vi "CSV SENDER 2 - Copy.vi"() -> ()   [LabVIEW 2021]
panel:
  out "Waveform Chart":dbl[](graph)
  out "Iteration terminal":i32
  in  "Stop 2":bool
  in  "File Path":path
  in  "Number of row to read \nat a time":i32=10000
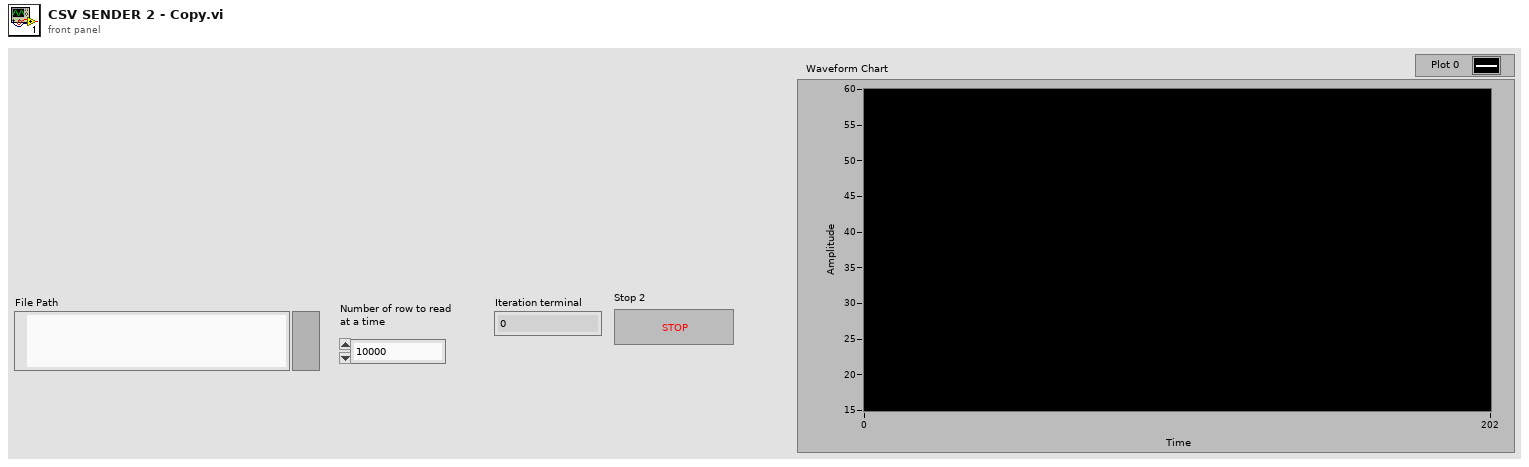
[diagram p1: front panel]
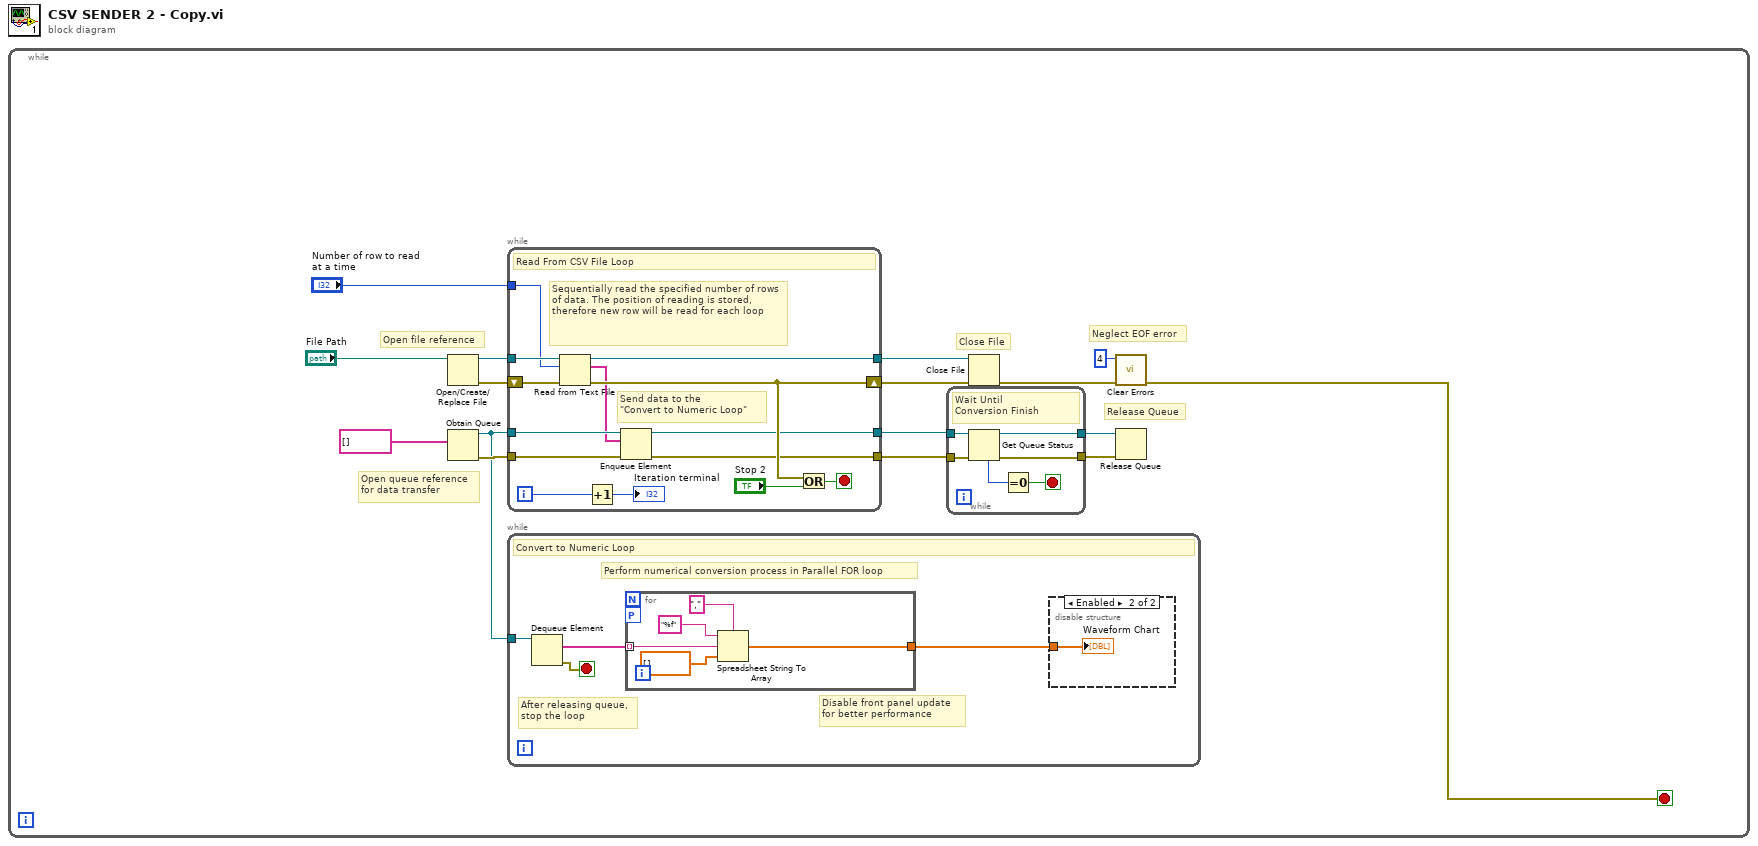
[diagram p0: block diagram]
diagram:
  n1 = while {
    stop <- w1 stop-if-true
    # "Neglect EOF error"
    # "Release Queue"
    # "Close File"
    # "Open queue reference\nfor data transfer"
    # "Open file reference"
    n2 = Open/Create/Replace File(file path (use dialog)="File Path") -> (refnum out=w14:refnum<file>, error out=w13:errorcluster)  [unwired: 5 in, 1 out]
    n3 = Obtain Queue(element data type=string[] [] ("形式文字列")) -> (queue out=w6:refnum<queue>, error out=w7:errorcluster)  [unwired: 4 in, 1 out]
    n4 = while {
      tunnel: w14 -> [w36]
      tunnel: [w34] -> w11
      shift-right: [w29] -> w10
      shift-left: w13 -> [w35]
      tunnel: "Number of row to read \nat a time" -> [w30]
      tunnel: w6 -> [w28]
      tunnel: w7 -> [w27]
      tunnel: [w25] -> w5
      tunnel: [w24] -> w4
      i -> [w32]
      stop <- w33 stop-if-true
      # "Send data to the \n\"Convert to Numeric Loop\""
      # "Sequentially read the specified number of rows of data. The position of reading is stored, therefore new row will be read for each loop"
      # "Read From CSV File Loop"
      n5 = Read from Text File(file (use dialog)=w36, count=w30, error in=w35) -> (refnum out=w34:refnum<file>, text=w26:string[], error out=w29:errorcluster)  [unwired: 1 in, 1 out]
      n6 = Increment(x=w32) -> (x+1=→"Iteration terminal":i32)
      n7 = Enqueue Element(queue=w28, element=w26, error in (no error)=w27) -> (queue out=w25:refnum<queue>, error out=w24:errorcluster)  [unwired: 1 in, 1 out]
      n8 = Or(x=w29, y="Stop 2") -> (x .or. y?=w33:bool)
    }
    n9 = while {
      tunnel: w6 -> [w40]
      stop <- w38 stop-if-true
      # "Disable front panel update \nfor better performance"
      # "After releasing queue,\nstop the loop"
      # "Perform numerical conversion process in Parallel FOR loop"
      # "Convert to Numeric Loop"
      n10 = Dequeue Element(queue=w40) -> (element=w39:string[], error out=w38:errorcluster)  [unwired: 2 in, 2 out]
      n11 = for "Forループ" {
        tunnel: w39 -> [w44] mode=indexing
        tunnel: [w42] -> w37
        workers-P: _ -> [_]
        n12 = Spreadsheet String To Array(delimiter (Tab)="," ("デリミタ（タブ）"), format string="%f" ("形式文字列"), spreadsheet string=w44, array type (2D Dbl)=dbl[] []) -> (array=w42:dbl[])
      }
      n13 = disable-structure shown="Enabled" {
        disable-tunnel: w37 -> [_ w41]
        frame Disabled {
        }
        frame Enabled {
          "Waveform Chart" <- w41
        }
      }
    }
    n14 = while {
      tunnel: w5 -> [w22]
      tunnel: w4 -> [w21]
      tunnel: [w18] -> w2
      tunnel: [w17] -> w3
      stop <- w19 stop-if-true
      # "Wait Until \nConversion Finish"
      n15 = Get Queue Status(queue=w22, error in (no error)=w21) -> (queue out=w18:refnum<queue>, error out=w17:errorcluster, # elements in queue=w20:i32)  [unwired: 1 in, 5 out]
      n16 = Equal To 0?(x=w20) -> (x = 0?=w19:bool)
    }
    n17 = Close File(refnum=w11, error in=w10) -> (error out=w9:errorcluster)  [unwired: 1 out]
    n18 = call <vilib>:"Clear Errors.vi"("error in (no error)"=w9, "specific error code to clear (0: all)"=4) -> ("error out"=w1:errorcluster)  [unwired: 4 in, 1 out]
    n19 = Release Queue(queue=w2, error in (no error)=w3) -> ()  [unwired: 1 in, 3 out]
  }
